vi "File Not Found Error Update.vi"(7 "Custom Message":string, 8 "error in":errorcluster, 11 "path in":path=path "c:/garbage") -> (0 "error out":errorcluster)   [LabVIEW 2021, in "File_CIF_U.lvlib"]
doc: "Many functions, such as the call library node, will provide error 7 but will not provide the path of the file that is missing. To simplify debugging, this will update the error message to provide the path of the missing file. If the original error did include the path this will strip it and replace it in the message. \nCustom Message can be used to prepend additional information in the error message such as what driver is missing on the system."
uses:
  File_CIF_U.lvlib
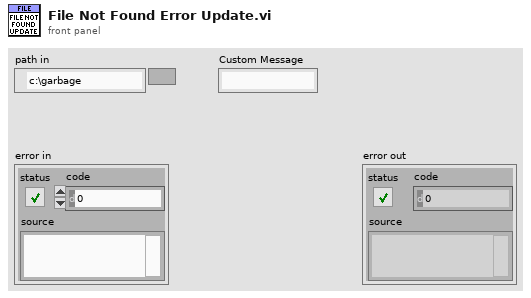
[diagram p1: front panel]
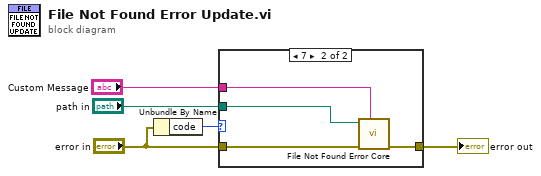
[diagram p0: block diagram]
diagram:
  n1 = Unbundle By Name("error in") -> ("code"=w5:i32)
  n2 = case shown="7" w5 {
    tunnel: "error in" -> [w6 w10]
    tunnel: [w6 w9] -> w3
    tunnel: "path in" -> [_ w8]
    tunnel: "Custom Message" -> [_ w7]
    frame 0, Default {
    }
    frame 7 {
      n3 = call "File Not Found Error Core.vi"("Custom Message"=w7, "error in"=w10, "path in"=w8) -> ("error out"=w9:errorcluster)  [unwired: 8 in]
    }
  }
  "error out" <- w3
